vi "BinaryDecodeDebug.vi"() -> ()   [LabVIEW 2010]
panel:
  out "Array":sgl[][](array[numeric]) format="%.3f"
  out "Bytes":u32
  in  "Received In":u8[](array[numeric])
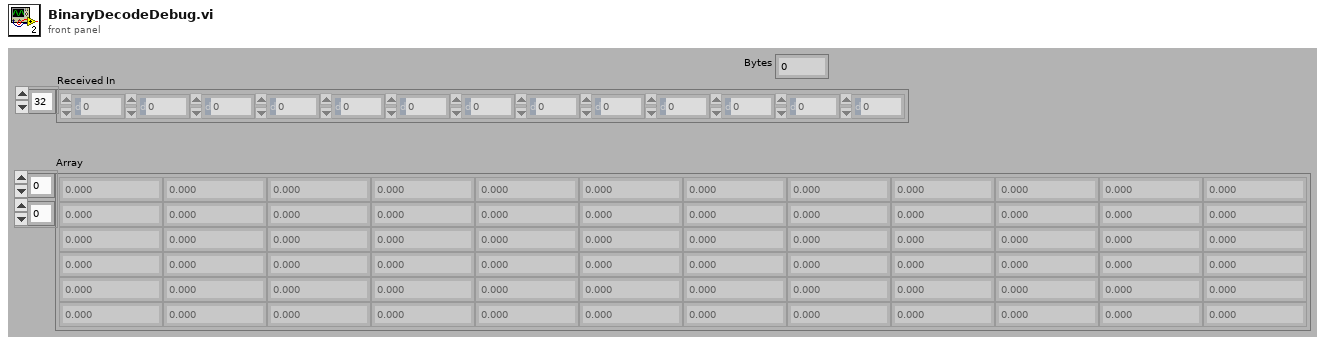
[diagram p1: front panel]
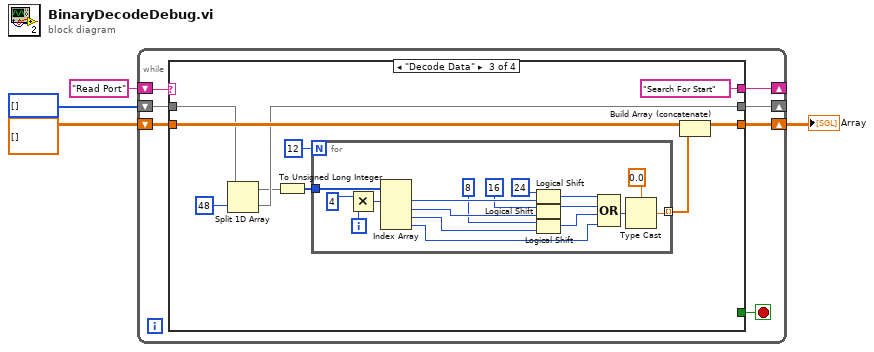
[diagram p0: block diagram]
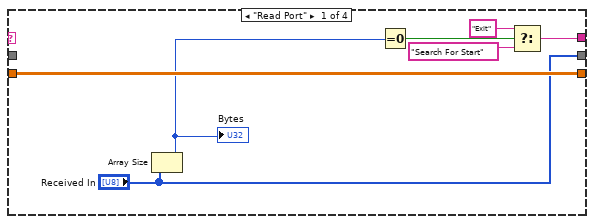
[diagram p2: hidden frame]
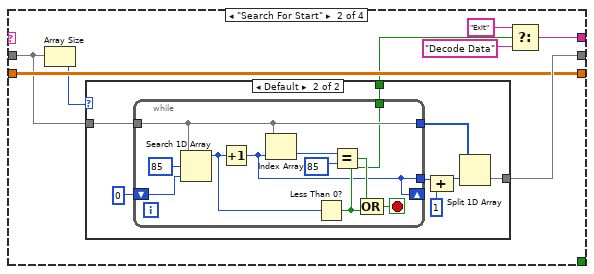
[diagram p3: hidden frame]
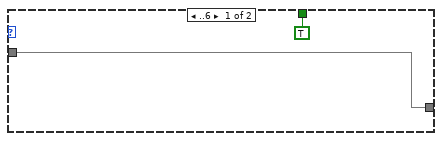
[diagram p4: hidden frame]
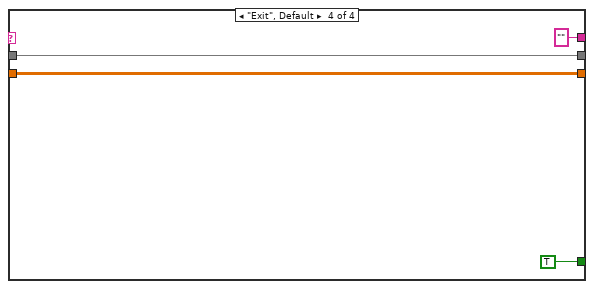
[diagram p5: hidden frame]
diagram:
  n1 = while {
    shift-right: [w9] -> _
    shift-left: "Read Port" ("t") -> [w11]
    shift-right: [w8] -> _
    shift-left: u8[] [] ("unsigned byte array") -> [w7]
    shift-right: [w5] -> w4
    shift-left: sgl[][] [] ("unsigned byte array") -> [w6]
    stop <- w10 stop-if-true
    n2 = case shown="\"Decode Data\"" w11 {
      tunnel: [_ _ _ TRUE] -> w10
      tunnel: [w14 w20 "Search For Start" ""] -> w9
      tunnel: ["Received In" w26 w51 w75] -> w8
      tunnel: w7 -> [_ w24 w53 w75]
      tunnel: w6 -> [w18 w25 w56 w74]
      tunnel: [w18 w25 w55 w74] -> w5
      frame "Read Port" {
        n3 = Array Size(array="Received In") -> (size(s)=w12:i32)
        "Bytes" <- w12
        n4 = Equal To 0?(x=w12) -> (x = 0?=w15:bool)
        n5 = Select(t="Exit", s=w15, f="Search For Start") -> (s? t:f=w14:string)
      }
      frame "Search For Start" {
        n6 = Array Size(array=w24) -> (size(s)=w23:i32)
        n7 = case shown="Default" w23 {
          tunnel: [w28 w35] -> w26
          tunnel: w24 -> [w28 w34]
          tunnel: [TRUE w30] -> w22
          frame ..6 {
          }
          frame Default {
            n8 = while {
              tunnel: [w37] -> w33
              tunnel: [w44] -> w36
              tunnel: w34 -> [w44]
              tunnel: [w39] -> w30
              shift-right: [w37] -> _
              shift-left: 0 -> [w38]
              stop <- w41 stop-if-true
              n9 = Search 1D Array(1D array=w44, element=u8 85, start index (0)=w38) -> (index of element=w40:i32)
              n10 = Increment(x=w40) -> (x+1=w37:i32)
              n11 = Index Array(array=w44, index=w37) -> (element=w45:u8)
              n12 = Less Than 0?(x=w40) -> (x < 0?=w39:bool)
              n13 = Equal?(x=w45, y=u8 85 ("element")) -> (x = y?=w42:bool)
              n14 = Compound Arithmetic op=OR(w42, w39) -> (w41:bool)
            }
            n15 = Compound Arithmetic op=ADD(w33, 1 ("value")) -> (w32:i32)
            n16 = Split 1D Array(array=w36, index=w32) -> (second subarray=w35:u8[])  [unwired: 1 out]
          }
        }
        n17 = Select(t="Exit", s=w22, f="Decode Data") -> (s? t:f=w20:string)
      }
      frame "Decode Data" {
        n18 = Split 1D Array(array=w53, index=48) -> (first subarray=w47:u8[], second subarray=w51:u8[])
        n19 = To Unsigned Long Integer(number=w47) -> (unsigned 32bit integer=w50:u32[])
        n20 = for {
          N: 12 -> [_]
          tunnel: w50 -> [w72]
          tunnel: [w57] -> w49 mode=indexing
          i -> [w61]
          n21 = Multiply(x=4, y=w61) -> (x*y=w62:i32)
          n22 = Index Array(array=w72, index #1=w62) -> (element #1=w73:u32, element #2=w70:u32, element #3=w69:u32, element #4=w63:u32)  [unwired: 3 in]
          n23 = Logical Shift(y=i16 24, x=w73) -> (x << y=w66:u32)
          n24 = Logical Shift(y=i16 16, x=w70) -> (x << y=w65:u32)
          n25 = Logical Shift(y=i16 8, x=w69) -> (x << y=w64:u32)
          n26 = Compound Arithmetic op=OR(w66, w65, w64, w63) -> (w58:u32)
          n27 = Type Cast(type=sgl 0.0, x=w58) -> (*(type *) &x=w57:sgl)
        }
        n28 = Build Array (concatenate)(w56, w49) -> (w55:sgl[][])
      }
      frame "Exit", Default {
      }
    }
  }
  "Array" <- w4
